vi "Read Shared Variable - General - Refnum - Ver 2.vi"(8 "Error In":errorcluster, 9 "Type code":i32, 10 "Variable Refnum":variant) -> (0 "Error Out":errorcluster, 1 "Data":variant, 2 "size(s)":i32[](array[numeric]), 3 "Size":string)   [LabVIEW 2014]
doc: "<B>Copyright</B>: (c) MHWirth 2015. All rights are reserved.\n\nThis SubVI reads the shared variable and returns it as a variant. It returns the size of the variable in two formats: numeric and string.\n\nSupported shared variable types:\nCode 1. Boolean\nCode 2 to 5. Int8/16/32/64\nCode 6 to 9. UInt8/16/32/64\nCode 10. Double\nCode 11. Single-precision\nCode 12. String\nCode 13-23 - 1D array of above types except string\n\n<B>Error 7001</B>: Unknown Data Type - Type Code Array (Int32) contains -1 indicating an unknown data type."
uses:
  Variable Refnum Cluster.ctl
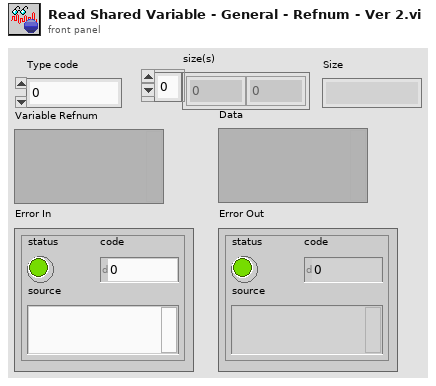
[diagram p1: front panel]
types:
  T1 = typedef "Variable Refnum Cluster.ctl" = cluster{"1":refnum<k21>, "2":refnum<k21>, "3":refnum<k21>, "4":refnum<k21>, "5":refnum<k21>, "6":refnum<k21>, "7":refnum<k21>, "8":refnum<k21>, "9":refnum<k21>, "10":refnum<k21>, "11":refnum<k21>, "12":refnum<k21>, "13":refnum<k21>, "14":refnum<k21>, "15":refnum<k21>, "16":refnum<k21>, "17":refnum<k21>, "18":refnum<k21>, "19":refnum<k21>, "20":refnum<k21>, "21":refnum<k21>, "22":refnum<k21>, "23":refnum<k21>, "24":refnum<k21>, "25":refnum<k21>, "26":refnum<k21>, "27":refnum<k21>, "28":refnum<k21>, "29":refnum<k21>, "30":refnum<k21>, "31":refnum<k21>, "32":refnum<k21>, "33":refnum<k21>, "34":refnum<k21>, "35":refnum<k21>, "36":refnum<k21>}
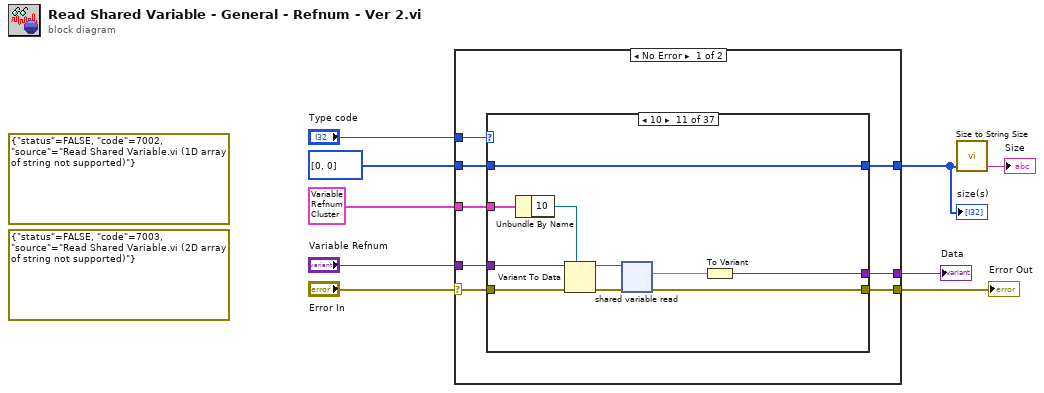
[diagram p0: block diagram]
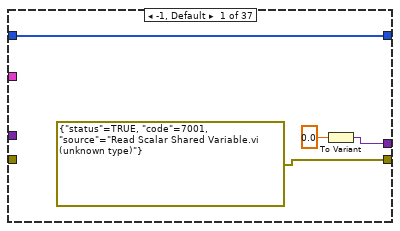
[diagram p2: hidden frame]
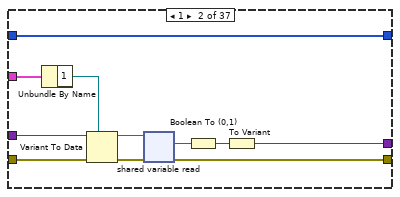
[diagram p3: hidden frame]
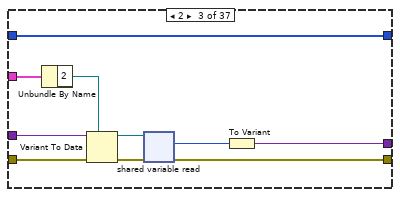
[diagram p4: hidden frame]
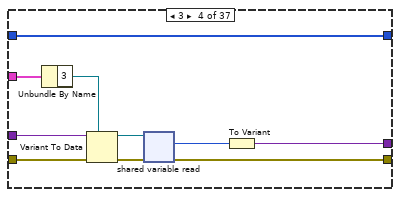
[diagram p5: hidden frame]
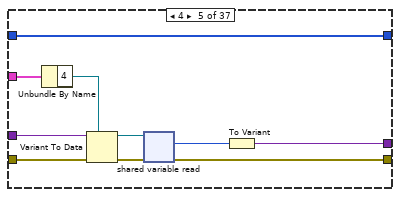
[diagram p6: hidden frame]
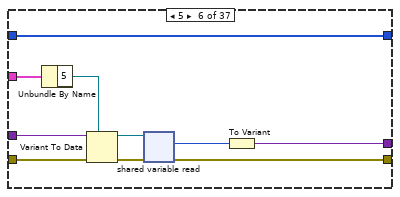
[diagram p7: hidden frame]
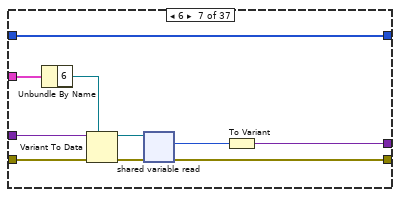
[diagram p8: hidden frame]
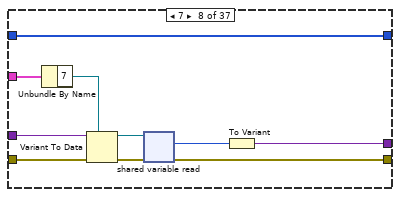
[diagram p9: hidden frame]
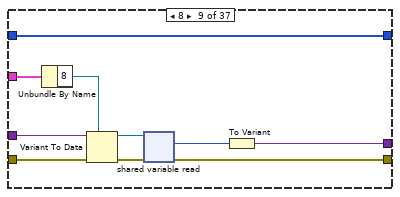
[diagram p10: hidden frame]
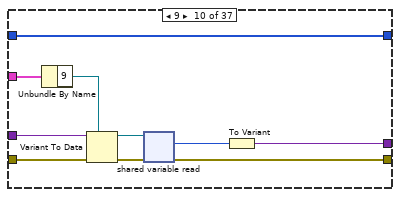
[diagram p11: hidden frame]
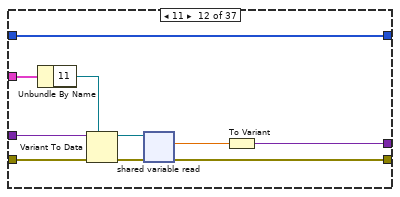
[diagram p12: hidden frame]
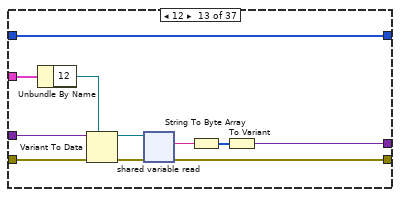
[diagram p13: hidden frame]
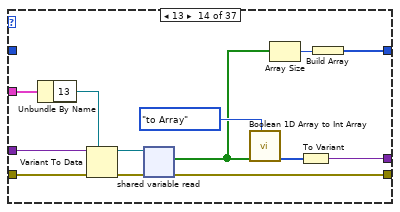
[diagram p14: hidden frame]
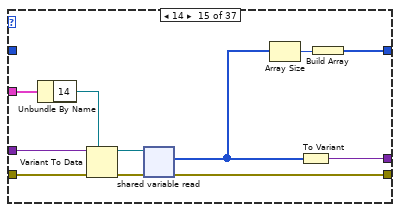
[diagram p15: hidden frame]
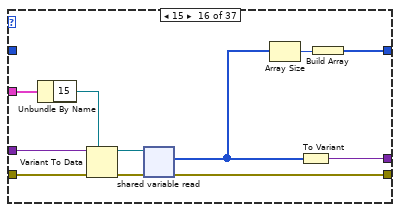
[diagram p16: hidden frame]
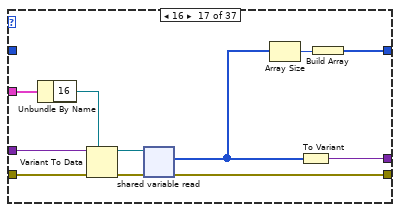
[diagram p17: hidden frame]
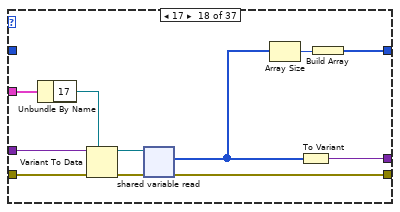
[diagram p18: hidden frame]
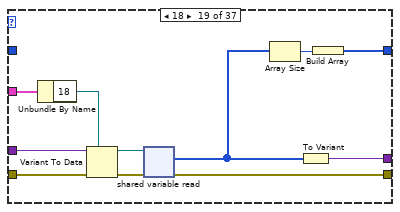
[diagram p19: hidden frame]
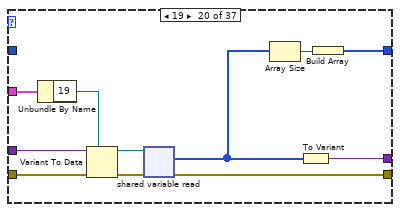
[diagram p20: hidden frame]
diagram:
  (unwired) errorcluster {"status"=FALSE, "code"=7002, "source"="Read Shared Variable.vi (1D array of string not supported)"} ("Error In")
  (unwired) errorcluster {"status"=FALSE, "code"=7003, "source"="Read Shared Variable.vi (2D array of string not supported)"} ("Error In")
  n1 = case shown="No Error" "Error In" {
    selector: "Error In" -> [w14 w400]
    tunnel: "Type code" -> [w17 _]
    tunnel: "Variable Refnum" -> [w16 w401]
    tunnel: T1 {"1"="", "2"="", "3"="", "4"="", "5"="", "6"="", "7"="", "8"="", "9"="", "10"="", "11"="", "12"="", "13"="", "14"="", "15"="", "16"="", "17"="", "18"="", "19"="", "20"="", "21"="", "22"="", "23"="", "24"="", "25"="", "26"="", "27"="", "28"="", "29"="", "30"="", "31"="", "32"="", "33"="", "34"="", "35"="", "36"=""} ("output cluster") -> [w15 _]
    tunnel: [w13 w401] -> w4
    tunnel: [w12 w400] -> w3
    tunnel: [w11 w402] -> w2
    tunnel: i32[] [0, 0] ("size(s)") -> [w10 w402]
    frame No Error {
      n2 = case shown="10" w17 {
        tunnel: w16 -> [_ w32 w42 w52 w62 w72 w82 w92 w102 w112 w122 w132 w143 w156 w167 w178 w189 w200 w211 w222 w233 w244 w255 w266 w277 w289 w299 w309 w319 w329 w339 w349 w359 w369 w379 w389 w399]
        tunnel: w15 -> [_ w31 w41 w51 w61 w71 w81 w91 w101 w111 w121 w131 w142 w155 w166 w177 w188 w199 w210 w221 w232 w243 w254 w265 w276 w288 w298 w308 w318 w328 w338 w348 w358 w368 w378 w388 w398]
        tunnel: w14 -> [_ w29 w39 w49 w59 w69 w79 w89 w99 w109 w119 w129 w140 w153 w164 w175 w186 w197 w208 w219 w230 w241 w252 w263 w274 w286 w296 w306 w316 w326 w336 w346 w356 w366 w376 w386 w396]
        tunnel: [w18 w24 w36 w46 w56 w66 w76 w86 w96 w106 w116 w126 w137 w150 w161 w172 w183 w194 w205 w216 w227 w238 w249 w260 w271 w283 w293 w303 w313 w323 w333 w343 w353 w363 w373 w383 w393] -> w13
        tunnel: [errorcluster {"status"=TRUE, "code"=7001, "source"="Read Scalar Shared Variable.vi (unknown type)"} ("error constant") w23 w35 w45 w55 w65 w75 w85 w95 w105 w115 w125 w136 w149 w160 w171 w182 w193 w204 w215 w226 w237 w248 w259 w270 w282 w292 w302 w312 w322 w332 w342 w352 w362 w372 w382 w392] -> w12
        tunnel: [w21 w22 w34 w44 w54 w64 w74 w84 w94 w104 w114 w124 w135 w144 w158 w169 w180 w191 w202 w213 w224 w235 w246 w257 w268 w278 w291 w301 w311 w321 w331 w341 w351 w361 w371 w381 w391] -> w11
        tunnel: w10 -> [w21 w22 w34 w44 w54 w64 w74 w84 w94 w104 w114 w124 w135 _ _ _ _ _ _ _ _ _ _ _ _ _ _ _ _ _ _ _ _ _ _ _ _]
        frame -1, Default {
          n3 = To Variant(anything=0.0) -> (Variant=w18:variant)
        }
        frame 1 {
          n4 = Unbundle By Name(w31) -> ("1"=w30:refnum<k21>)
          n5 = Variant To Data(error in=w29, type=w30, Variant=w32) -> (data=w28:refnum<k21>, error out=w27:errorcluster)
          n6 = shared-variable-read(w28, w27) -> (w23:errorcluster, w26:bool)  [unwired: 2 out]
          n7 = Boolean To (0,1)(Boolean=w26) -> (0, 1=w25:i16)
          n8 = To Variant(anything=w25) -> (Variant=w24:variant)
        }
        frame 2 {
          n9 = Unbundle By Name(w41) -> ("2"=w40:refnum<k21>)
          n10 = Variant To Data(error in=w39, type=w40, Variant=w42) -> (data=w38:refnum<k21>, error out=w37:errorcluster)
          n11 = shared-variable-read(w38, w37) -> (w35:errorcluster, w33:i8)  [unwired: 2 out]
          n12 = To Variant(anything=w33) -> (Variant=w36:variant)
        }
        frame 3 {
          n13 = Unbundle By Name(w51) -> ("3"=w50:refnum<k21>)
          n14 = Variant To Data(error in=w49, type=w50, Variant=w52) -> (data=w48:refnum<k21>, error out=w47:errorcluster)
          n15 = shared-variable-read(w48, w47) -> (w45:errorcluster, w43:i16)  [unwired: 2 out]
          n16 = To Variant(anything=w43) -> (Variant=w46:variant)
        }
        frame 4 {
          n17 = Unbundle By Name(w61) -> ("4"=w60:refnum<k21>)
          n18 = Variant To Data(error in=w59, type=w60, Variant=w62) -> (data=w58:refnum<k21>, error out=w57:errorcluster)
          n19 = shared-variable-read(w58, w57) -> (w55:errorcluster, w53:i32)  [unwired: 2 out]
          n20 = To Variant(anything=w53) -> (Variant=w56:variant)
        }
        frame 5 {
          n21 = Unbundle By Name(w71) -> ("5"=w70:refnum<k21>)
          n22 = Variant To Data(error in=w69, type=w70, Variant=w72) -> (data=w68:refnum<k21>, error out=w67:errorcluster)
          n23 = shared-variable-read(w68, w67) -> (w65:errorcluster, w63:i64)  [unwired: 2 out]
          n24 = To Variant(anything=w63) -> (Variant=w66:variant)
        }
        frame 6 {
          n25 = Unbundle By Name(w81) -> ("6"=w80:refnum<k21>)
          n26 = Variant To Data(error in=w79, type=w80, Variant=w82) -> (data=w78:refnum<k21>, error out=w77:errorcluster)
          n27 = shared-variable-read(w78, w77) -> (w75:errorcluster, w73:u8)  [unwired: 2 out]
          n28 = To Variant(anything=w73) -> (Variant=w76:variant)
        }
        frame 7 {
          n29 = Unbundle By Name(w91) -> ("7"=w90:refnum<k21>)
          n30 = Variant To Data(error in=w89, type=w90, Variant=w92) -> (data=w88:refnum<k21>, error out=w87:errorcluster)
          n31 = shared-variable-read(w88, w87) -> (w85:errorcluster, w83:u16)  [unwired: 2 out]
          n32 = To Variant(anything=w83) -> (Variant=w86:variant)
        }
        frame 8 {
          n33 = Unbundle By Name(w101) -> ("8"=w100:refnum<k21>)
          n34 = Variant To Data(error in=w99, type=w100, Variant=w102) -> (data=w98:refnum<k21>, error out=w97:errorcluster)
          n35 = shared-variable-read(w98, w97) -> (w95:errorcluster, w93:u32)  [unwired: 2 out]
          n36 = To Variant(anything=w93) -> (Variant=w96:variant)
        }
        frame 9 {
          n37 = Unbundle By Name(w111) -> ("9"=w110:refnum<k21>)
          n38 = Variant To Data(error in=w109, type=w110, Variant=w112) -> (data=w108:refnum<k21>, error out=w107:errorcluster)
          n39 = shared-variable-read(w108, w107) -> (w105:errorcluster, w103:u64)  [unwired: 2 out]
          n40 = To Variant(anything=w103) -> (Variant=w106:variant)
        }
        frame 10 {
          n41 = Unbundle By Name(w121) -> ("10"=w120:refnum<k21>)
          n42 = Variant To Data(error in=w119, type=w120, Variant=w122) -> (data=w118:refnum<k21>, error out=w117:errorcluster)
          n43 = shared-variable-read(w118, w117) -> (w115:errorcluster, w113:dbl)  [unwired: 2 out]
          n44 = To Variant(anything=w113) -> (Variant=w116:variant)
        }
        frame 11 {
          n45 = Unbundle By Name(w131) -> ("11"=w130:refnum<k21>)
          n46 = Variant To Data(error in=w129, type=w130, Variant=w132) -> (data=w128:refnum<k21>, error out=w127:errorcluster)
          n47 = shared-variable-read(w128, w127) -> (w125:errorcluster, w123:sgl)  [unwired: 2 out]
          n48 = To Variant(anything=w123) -> (Variant=w126:variant)
        }
        frame 12 {
          n49 = Unbundle By Name(w142) -> ("12"=w141:refnum<k21>)
          n50 = Variant To Data(error in=w140, type=w141, Variant=w143) -> (data=w139:refnum<k21>, error out=w138:errorcluster)
          n51 = shared-variable-read(w139, w138) -> (w136:errorcluster, w134:string)  [unwired: 2 out]
          n52 = String To Byte Array(string=w134) -> (unsigned byte array=w133:u8[])
          n53 = To Variant(anything=w133) -> (Variant=w137:variant)
        }
        frame 13 {
          n54 = Unbundle By Name(w155) -> ("13"=w154:refnum<k21>)
          n55 = Variant To Data(error in=w153, type=w154, Variant=w156) -> (data=w152:refnum<k21>, error out=w151:errorcluster)
          n56 = shared-variable-read(w152, w151) -> (w149:errorcluster, w146:bool[])  [unwired: 2 out]
          n57 = call "Boolean 1D Array to Int Array.vi"("Mode"=enum16{"to Array", "to Number"}."to Array" ("Enum"), "Array of Boolean"=w146) -> ("Array out"=w148:u32[])  [unwired: 8 in]
          n58 = Array Size(array=w146) -> (size(s)=w145:i32)
          n59 = To Variant(anything=w148) -> (Variant=w150:variant)
          n60 = Build Array(w145) -> (w144:i32[])
        }
        frame 14 {
          n61 = Unbundle By Name(w166) -> ("14"=w165:refnum<k21>)
          n62 = Variant To Data(error in=w164, type=w165, Variant=w167) -> (data=w163:refnum<k21>, error out=w162:errorcluster)
          n63 = shared-variable-read(w163, w162) -> (w160:errorcluster, w157:i8[])  [unwired: 2 out]
          n64 = Array Size(array=w157) -> (size(s)=w159:i32)
          n65 = To Variant(anything=w157) -> (Variant=w161:variant)
          n66 = Build Array(w159) -> (w158:i32[])
        }
        frame 15 {
          n67 = Unbundle By Name(w177) -> ("15"=w176:refnum<k21>)
          n68 = Variant To Data(error in=w175, type=w176, Variant=w178) -> (data=w174:refnum<k21>, error out=w173:errorcluster)
          n69 = shared-variable-read(w174, w173) -> (w171:errorcluster, w168:i16[])  [unwired: 2 out]
          n70 = Array Size(array=w168) -> (size(s)=w170:i32)
          n71 = To Variant(anything=w168) -> (Variant=w172:variant)
          n72 = Build Array(w170) -> (w169:i32[])
        }
        frame 16 {
          n73 = Unbundle By Name(w188) -> ("16"=w187:refnum<k21>)
          n74 = Variant To Data(error in=w186, type=w187, Variant=w189) -> (data=w185:refnum<k21>, error out=w184:errorcluster)
          n75 = shared-variable-read(w185, w184) -> (w182:errorcluster, w179:i32[])  [unwired: 2 out]
          n76 = Array Size(array=w179) -> (size(s)=w181:i32)
          n77 = To Variant(anything=w179) -> (Variant=w183:variant)
          n78 = Build Array(w181) -> (w180:i32[])
        }
        frame 17 {
          n79 = Unbundle By Name(w199) -> ("17"=w198:refnum<k21>)
          n80 = Variant To Data(error in=w197, type=w198, Variant=w200) -> (data=w196:refnum<k21>, error out=w195:errorcluster)
          n81 = shared-variable-read(w196, w195) -> (w193:errorcluster, w190:i64[])  [unwired: 2 out]
          n82 = Array Size(array=w190) -> (size(s)=w192:i32)
          n83 = To Variant(anything=w190) -> (Variant=w194:variant)
          n84 = Build Array(w192) -> (w191:i32[])
        }
        frame 18 {
          n85 = Unbundle By Name(w210) -> ("18"=w209:refnum<k21>)
          n86 = Variant To Data(error in=w208, type=w209, Variant=w211) -> (data=w207:refnum<k21>, error out=w206:errorcluster)
          n87 = shared-variable-read(w207, w206) -> (w204:errorcluster, w201:u8[])  [unwired: 2 out]
          n88 = Array Size(array=w201) -> (size(s)=w203:i32)
          n89 = To Variant(anything=w201) -> (Variant=w205:variant)
          n90 = Build Array(w203) -> (w202:i32[])
        }
        frame 19 {
          n91 = Unbundle By Name(w221) -> ("19"=w220:refnum<k21>)
          n92 = Variant To Data(error in=w219, type=w220, Variant=w222) -> (data=w218:refnum<k21>, error out=w217:errorcluster)
          n93 = shared-variable-read(w218, w217) -> (w215:errorcluster, w212:u16[])  [unwired: 2 out]
          n94 = Array Size(array=w212) -> (size(s)=w214:i32)
          n95 = To Variant(anything=w212) -> (Variant=w216:variant)
          n96 = Build Array(w214) -> (w213:i32[])
        }
        frame 20 {
          n97 = Unbundle By Name(w232) -> ("20"=w231:refnum<k21>)
          n98 = Variant To Data(error in=w230, type=w231, Variant=w233) -> (data=w229:refnum<k21>, error out=w228:errorcluster)
          n99 = shared-variable-read(w229, w228) -> (w226:errorcluster, w223:u32[])  [unwired: 2 out]
          n100 = Array Size(array=w223) -> (size(s)=w225:i32)
          n101 = To Variant(anything=w223) -> (Variant=w227:variant)
          n102 = Build Array(w225) -> (w224:i32[])
        }
        frame 21 {
          n103 = Unbundle By Name(w243) -> ("21"=w242:refnum<k21>)
          n104 = Variant To Data(error in=w241, type=w242, Variant=w244) -> (data=w240:refnum<k21>, error out=w239:errorcluster)
          n105 = shared-variable-read(w240, w239) -> (w237:errorcluster, w234:u64[])  [unwired: 2 out]
          n106 = Array Size(array=w234) -> (size(s)=w236:i32)
          n107 = To Variant(anything=w234) -> (Variant=w238:variant)
          n108 = Build Array(w236) -> (w235:i32[])
        }
        frame 22 {
          n109 = Unbundle By Name(w254) -> ("22"=w253:refnum<k21>)
          n110 = Variant To Data(error in=w252, type=w253, Variant=w255) -> (data=w251:refnum<k21>, error out=w250:errorcluster)
          n111 = shared-variable-read(w251, w250) -> (w248:errorcluster, w245:dbl[])  [unwired: 2 out]
          n112 = Array Size(array=w245) -> (size(s)=w247:i32)
          n113 = To Variant(anything=w245) -> (Variant=w249:variant)
          n114 = Build Array(w247) -> (w246:i32[])
        }
        frame 23 {
          n115 = Unbundle By Name(w265) -> ("23"=w264:refnum<k21>)
          n116 = Variant To Data(error in=w263, type=w264, Variant=w266) -> (data=w262:refnum<k21>, error out=w261:errorcluster)
          n117 = shared-variable-read(w262, w261) -> (w259:errorcluster, w256:sgl[])  [unwired: 2 out]
          n118 = Array Size(array=w256) -> (size(s)=w258:i32)
          n119 = To Variant(anything=w256) -> (Variant=w260:variant)
          n120 = Build Array(w258) -> (w257:i32[])
        }
        frame 24 {
          n121 = Unbundle By Name(w276) -> ("24"=w275:refnum<k21>)
          n122 = Variant To Data(error in=w274, type=w275, Variant=w277) -> (data=w273:refnum<k21>, error out=w272:errorcluster)
          n123 = shared-variable-read(w273, w272) -> (w270:errorcluster, w267:string[])  [unwired: 2 out]
          n124 = Array Size(array=w267) -> (size(s)=w269:i32)
          n125 = To Variant(anything=w267) -> (Variant=w271:variant)
          n126 = Build Array(w269) -> (w268:i32[])
        }
        frame 25 {
          n127 = Unbundle By Name(w288) -> ("25"=w287:refnum<k21>)
          n128 = Variant To Data(error in=w286, type=w287, Variant=w289) -> (data=w285:refnum<k21>, error out=w284:errorcluster)
          n129 = shared-variable-read(w285, w284) -> (w282:errorcluster, w281:bool[][])  [unwired: 2 out]
          n130 = call "Boolean 2D Array to Int Array.vi"("Mode"=enum16{"to Array", "to Number"}."to Array" ("Enum"), "Array of Boolean"=w281) -> ("Array out"=w280:u32[][])  [unwired: 8 in]
          n131 = Array Size(array=w281) -> (size(s)=w278:i32[])
          n132 = To Variant(anything=w280) -> (Variant=w283:variant)
        }
        frame 26 {
          n133 = Unbundle By Name(w298) -> ("26"=w297:refnum<k21>)
          n134 = Variant To Data(error in=w296, type=w297, Variant=w299) -> (data=w295:refnum<k21>, error out=w294:errorcluster)
          n135 = shared-variable-read(w295, w294) -> (w292:errorcluster, w290:i8[][])  [unwired: 2 out]
          n136 = Array Size(array=w290) -> (size(s)=w291:i32[])
          n137 = To Variant(anything=w290) -> (Variant=w293:variant)
        }
        frame 27 {
          n138 = Unbundle By Name(w308) -> ("27"=w307:refnum<k21>)
          n139 = Variant To Data(error in=w306, type=w307, Variant=w309) -> (data=w305:refnum<k21>, error out=w304:errorcluster)
          n140 = shared-variable-read(w305, w304) -> (w302:errorcluster, w300:i16[][])  [unwired: 2 out]
          n141 = Array Size(array=w300) -> (size(s)=w301:i32[])
          n142 = To Variant(anything=w300) -> (Variant=w303:variant)
        }
        frame 28 {
          n143 = Unbundle By Name(w318) -> ("28"=w317:refnum<k21>)
          n144 = Variant To Data(error in=w316, type=w317, Variant=w319) -> (data=w315:refnum<k21>, error out=w314:errorcluster)
          n145 = shared-variable-read(w315, w314) -> (w312:errorcluster, w310:i32[][])  [unwired: 2 out]
          n146 = Array Size(array=w310) -> (size(s)=w311:i32[])
          n147 = To Variant(anything=w310) -> (Variant=w313:variant)
        }
        frame 29 {
          n148 = Unbundle By Name(w328) -> ("29"=w327:refnum<k21>)
          n149 = Variant To Data(error in=w326, type=w327, Variant=w329) -> (data=w325:refnum<k21>, error out=w324:errorcluster)
          n150 = shared-variable-read(w325, w324) -> (w322:errorcluster, w320:i64[][])  [unwired: 2 out]
          n151 = Array Size(array=w320) -> (size(s)=w321:i32[])
          n152 = To Variant(anything=w320) -> (Variant=w323:variant)
        }
        frame 30 {
          n153 = Unbundle By Name(w338) -> ("30"=w337:refnum<k21>)
          n154 = Variant To Data(error in=w336, type=w337, Variant=w339) -> (data=w335:refnum<k21>, error out=w334:errorcluster)
          n155 = shared-variable-read(w335, w334) -> (w332:errorcluster, w330:u8[][])  [unwired: 2 out]
          n156 = Array Size(array=w330) -> (size(s)=w331:i32[])
          n157 = To Variant(anything=w330) -> (Variant=w333:variant)
        }
        frame 31 {
          n158 = Unbundle By Name(w348) -> ("31"=w347:refnum<k21>)
          n159 = Variant To Data(error in=w346, type=w347, Variant=w349) -> (data=w345:refnum<k21>, error out=w344:errorcluster)
          n160 = shared-variable-read(w345, w344) -> (w342:errorcluster, w340:u16[][])  [unwired: 2 out]
          n161 = Array Size(array=w340) -> (size(s)=w341:i32[])
          n162 = To Variant(anything=w340) -> (Variant=w343:variant)
        }
        frame 32 {
          n163 = Unbundle By Name(w358) -> ("32"=w357:refnum<k21>)
          n164 = Variant To Data(error in=w356, type=w357, Variant=w359) -> (data=w355:refnum<k21>, error out=w354:errorcluster)
          n165 = shared-variable-read(w355, w354) -> (w352:errorcluster, w350:u32[][])  [unwired: 2 out]
          n166 = Array Size(array=w350) -> (size(s)=w351:i32[])
          n167 = To Variant(anything=w350) -> (Variant=w353:variant)
        }
        frame 33 {
          n168 = Unbundle By Name(w368) -> ("33"=w367:refnum<k21>)
          n169 = Variant To Data(error in=w366, type=w367, Variant=w369) -> (data=w365:refnum<k21>, error out=w364:errorcluster)
          n170 = shared-variable-read(w365, w364) -> (w362:errorcluster, w360:u64[][])  [unwired: 2 out]
          n171 = Array Size(array=w360) -> (size(s)=w361:i32[])
          n172 = To Variant(anything=w360) -> (Variant=w363:variant)
        }
        frame 34 {
          n173 = Unbundle By Name(w378) -> ("34"=w377:refnum<k21>)
          n174 = Variant To Data(error in=w376, type=w377, Variant=w379) -> (data=w375:refnum<k21>, error out=w374:errorcluster)
          n175 = shared-variable-read(w375, w374) -> (w372:errorcluster, w370:dbl[][])  [unwired: 2 out]
          n176 = Array Size(array=w370) -> (size(s)=w371:i32[])
          n177 = To Variant(anything=w370) -> (Variant=w373:variant)
        }
        frame 35 {
          n178 = Unbundle By Name(w388) -> ("35"=w387:refnum<k21>)
          n179 = Variant To Data(error in=w386, type=w387, Variant=w389) -> (data=w385:refnum<k21>, error out=w384:errorcluster)
          n180 = shared-variable-read(w385, w384) -> (w382:errorcluster, w380:sgl[][])  [unwired: 2 out]
          n181 = Array Size(array=w380) -> (size(s)=w381:i32[])
          n182 = To Variant(anything=w380) -> (Variant=w383:variant)
        }
        frame 36 {
          n183 = Unbundle By Name(w398) -> ("36"=w397:refnum<k21>)
          n184 = Variant To Data(error in=w396, type=w397, Variant=w399) -> (data=w395:refnum<k21>, error out=w394:errorcluster)
          n185 = shared-variable-read(w395, w394) -> (w392:errorcluster, w390:string[][])  [unwired: 2 out]
          n186 = Array Size(array=w390) -> (size(s)=w391:i32[])
          n187 = To Variant(anything=w390) -> (Variant=w393:variant)
        }
      }
    }
    frame Error {
    }
  }
  "Error Out" <- w3
  "size(s)" <- w2
  "Data" <- w4
  n188 = call "Size to String Size.vi"("size(s)"=w2) -> ("Size"=→"Size":string)  [unwired: 4 in]
